vi "MAIN - Acquire Data2.vi"() -> ()   [LabVIEW 2015]
uses:
  <vilib>/Platform/TimedLoop/XDataNode/timing_clust.ctl
  <vilib>/Platform/TimedLoop/XDataNode/nitl_modes.ctl
  <vilib>/Platform/TimedLoop/XDataNode/wakeup.ctl
  <vilib>/Platform/TimedLoop/XDataNode/XDataNode.xnode
  <vilib>/Platform/TimedLoop/XDataNode/XDNodeRunTimeDep.lvlib
panel:
  out "Current Free Space (Mb)":dbl
  out "Low on Free Disk Space":bool
  in  "Save Type":u16(ring) items=["USB", "cRIO"]
  out "Buffer":dbl(slide) scale=0.0..1.0
  in  "Buffer Size":u32=1000
  out "timed out?":bool
  out "ticks in":u32
  out "Waveform Graph":dbl[][](graph)
  out "ticks out":u32
  out "Error":errorcluster
  in  "Record":bool
  in  "Filename":string="default.txt"
  in  "Stop":bool
  in  "Sampling Freq [Hz]":dbl=200.0
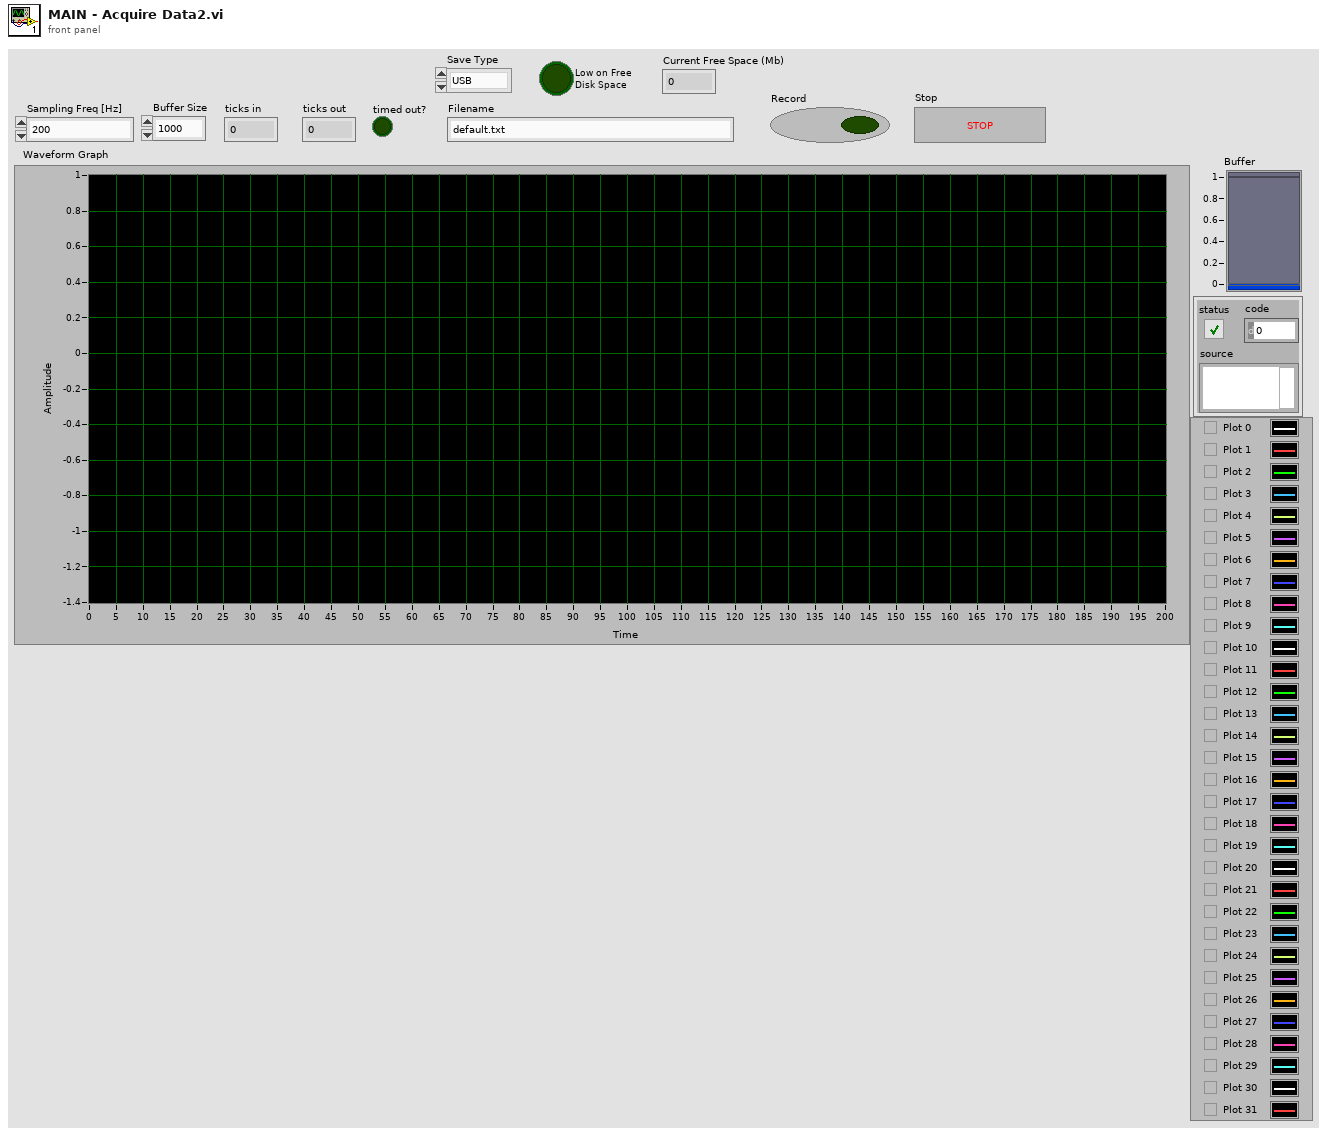
[diagram p1: front panel]
types:
  T1 = typedef "XDNodeRunTimeDep.lvlib/timing_clust.ctl" = cluster{"Expected End [f-1]":u64, "Actual End [f-1]":u64, "Finished Late? [f-1]":bool, "Expected End [i-1]":u64, "Actual End [i-1]":u64, "Finished Late? [i-1]":bool, "Expected Start [i]":u64, "Actual Start [i]":u64, "Expected Start [f]":u64, "Actual Start [f]":u64, "Source Name":string, "Structure Name":string, "Period":i64, "Deadline":i64, "Offset":i64, "Start":i64, "Priority":i32, "Timeout":i32, "Mode":T2, "Wakeup Reason":T3, "Error":errorcluster, "Source Type":string, "Secondary Source Type":string, "Global End Time":u64, "Global Start Time":u64, "Frame Duration":u64, "Iteration Duration":u64, "Assigned CPU":i32, "I/O Scan Engine Mode":u32}
  T2 = typedef "XDNodeRunTimeDep.lvlib/nitl_modes.ctl" = enum32{"No Change", "Process missed periods, maintain original phase", "Discard missed periods, maintain original phase", "Process missed periods, ignore original phase", "Discard missed periods, ignore original phase"}
  T3 = typedef "XDNodeRunTimeDep.lvlib/wakeup.ctl" = enum32{"Normal", "Aborted", "Asynchronous wakeup", "Timing source error", "Timed loop error", "Timeout"}
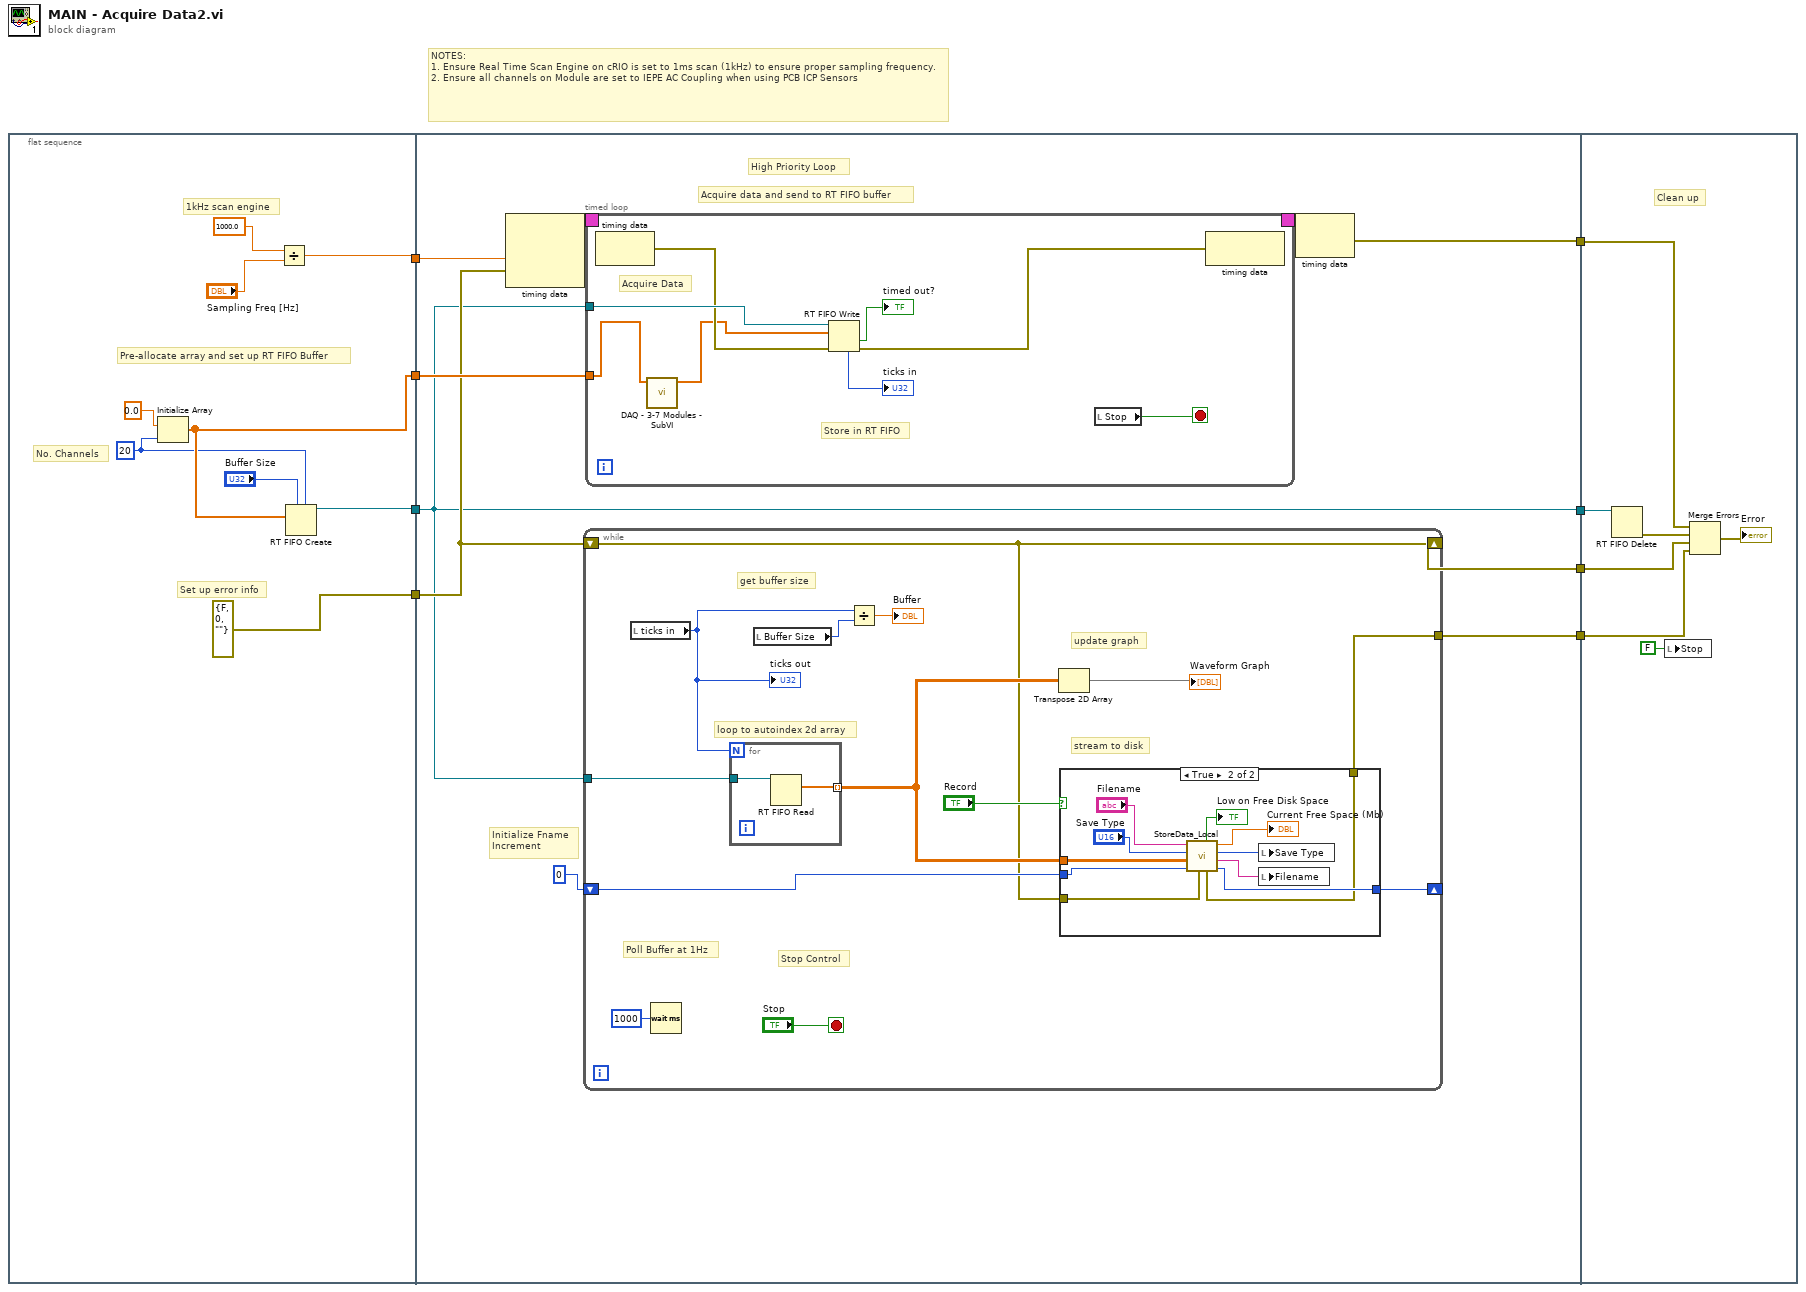
[diagram p0: block diagram]
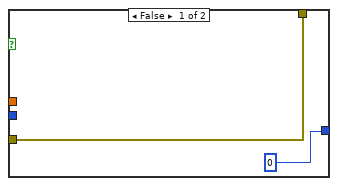
[diagram p2: hidden frame]
diagram:
  # "NOTES:\n1. Ensure Real Time Scan Engine on cRIO is set to 1ms scan (1kHz) to ensure proper sampling frequency.\n2. Ensure all channels on Module are set to IEPE AC Coupling when using PCB ICP Sensors"
  n1 = flat-sequence {
    tunnel: [w12] -> w8
    tunnel: [w17] -> w7
    tunnel: [w14] -> w6
    tunnel: [errorcluster {"status"=FALSE, "code"=0, "source"=""} ("Error")] -> w5
    tunnel: w8 -> [w25]
    tunnel: w7 -> [w24]
    tunnel: w6 -> [w20]
    tunnel: w5 -> [w23]
    tunnel: [w22] -> w4
    tunnel: [w21] -> w3
    tunnel: [w20] -> w2
    tunnel: [w19] -> w1
    tunnel: w4 -> [w81]
    tunnel: w3 -> [w76]
    tunnel: w2 -> [w78]
    tunnel: w1 -> [w75]
    frame #0 {
      w10 = 20 ("dimension size")
      # "No. Channels"
      # "Pre-allocate array and set up RT FIFO Buffer"
      # "1kHz scan engine"
      # "Set up error info"
      n2 = Initialize Array(0.0 ("element"), w10) -> (w12:dbl[])
      n3 = Divide(x=1000.0, y="Sampling Freq [Hz]") -> (x/y=w17:dbl)
      n4 = RT FIFO Create(1:w12, 4:"Buffer Size", 6:w10) -> (8:w14:refnum<k33>)  [unwired: 5 in, 2 out]
    }
    frame #1 {
      # "Initialize Fname \nIncrement"
      # "Acquire data and send to RT FIFO buffer"
      # "High Priority Loop"
      n5 = node-c288(w24, w23) -> (w27:T1)  [unwired: 1 in]
      n6 = while {
        tunnel: w20 -> [w39]
        shift-right: [w28] -> w21
        shift-left: w23 -> [w28]
        tunnel: [w31] -> w19
        shift-right: [w29] -> _
        shift-left: u8 0 -> [w30]
        stop <- "Stop" stop-if-true
        # "stream to disk"
        # "Stop Control"
        # "get buffer size"
        # "Poll Buffer at 1Hz"
        # "loop to autoindex 2d array"
        # "update graph"
        n7 = local read "ticks in"() -> (w33:u32)
        "ticks out" <- w33
        n8 = Wait (ms)(milliseconds to wait=u32 1000) -> ()  [unwired: 1 out]
        n9 = for {
          N: w33 -> [_]
          tunnel: [w42] -> w38 mode=indexing
          tunnel: w39 -> [w41]
          n10 = RT FIFO Read(0:w41) -> (9:w42:dbl[])  [unwired: 3 in, 4 out]
        }
        n11 = local read "Buffer Size"() -> (w32:u32)
        n12 = Divide(x=w33, y=w32) -> (x/y=→"Buffer":dbl)
        n13 = Transpose 2D Array(2D array=w38) -> (transposed array=→"Waveform Graph":dbl[][])
        n14 = case shown="True" "Record" {
          tunnel: w38 -> [_ w55]
          tunnel: [w43 w48] -> w31
          tunnel: w30 -> [_ w50]
          tunnel: [u8 0 w49] -> w29
          tunnel: w28 -> [w43 w45]
          frame False {
          }
          frame True {
            n15 = call "StoreData_Local.vi"("error in (no error)"=w45, "Fname Increment"=w50, "Array"=w55, "Save Type"="Save Type", "Filename"="Filename") -> ("NewFnameCount"=w49:u8, "New Fname"=w46:string, "New Save Type"=w47:u16, "Current Free Space (Mb)"=→"Current Free Space (Mb)":dbl, "error out"=w48:errorcluster, "Low on Free Disk Space"=→"Low on Free Disk Space":bool)  [unwired: 1 in]
            n16 = local write "Save Type"(w47) -> ()
            n17 = local write "Filename"(w46) -> ()
          }
        }
      }
      n18 = timed-loop {
        timing: w27 -> [_]
        timing-out: [_] -> w26
        tunnel: w25 -> [w57]
        tunnel: w20 -> [w63]
        stop <- w58 stop-if-true
        # "Store in RT FIFO"
        # "Acquire Data"
        n19 = node-c288() -> (w62:errorcluster)  [unwired: 1 in]
        n20 = call "DAQ - 3-7 Modules - SubVI.vi"("array"=w57) -> ("output array"=w56:dbl[])  [unwired: 10 in]
        n21 = RT FIFO Write(0:w63, 1:w56, 3:w62) -> (7:→"ticks in":u32, 10:→"timed out?":bool, 11:w61:errorcluster)  [unwired: 2 in, 1 out]
        n22 = local read "Stop"() -> (w58:bool)
        n23 = node-c288(w61) -> ()  [unwired: 1 out]
      }
      n24 = node-c288(w26) -> (w22:errorcluster)
    }
    frame #2 {
      # "Clean up"
      n25 = RT FIFO Delete(0:w78) -> (11:w77:errorcluster)  [unwired: 2 in]
      n26 = local write "Stop"(FALSE ("Stop")) -> ()
      n27 = Merge Errors(w81, w77, w76, w75) -> (→"Error":errorcluster)
    }
  }
